vi "4.CVT Basic Writer.vi"() -> ()   [LabVIEW 2014]
uses:
  vi.lib/Q-WaveSystems/QwaveSys Raspberry Pi for LabVIEW Home-Education/CVT/_SubVIs/TypeDefs/cvt_Tag Configuration.ctl
  vi.lib/Q-WaveSystems/QwaveSys Raspberry Pi for LabVIEW Home-Education/CVT/_SubVIs/TypeDefs/cvt_Data Types.ctl
  vi.lib/Q-WaveSystems/QwaveSys Raspberry Pi for LabVIEW Home-Education/QwaveSys Raspberry Pi Library.lvlib
panel:
  out "Variable Name":string
  in  "stop":bool
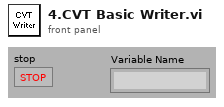
[diagram p1: front panel]
types:
  T1 = typedef "QwaveSys Raspberry Pi Library.lvlib/cvt_Tag Configuration.ctl" = cluster{"Name":string, "Data Type":T2, "Array":bool, "Size":u32, "Default":string, "Enum":string[], "Description":string}
  T2 = typedef "QwaveSys Raspberry Pi Library.lvlib/cvt_Data Types.ctl" = enum16{"Bool", "U8", "I32", "Double", "String", "Enum"}
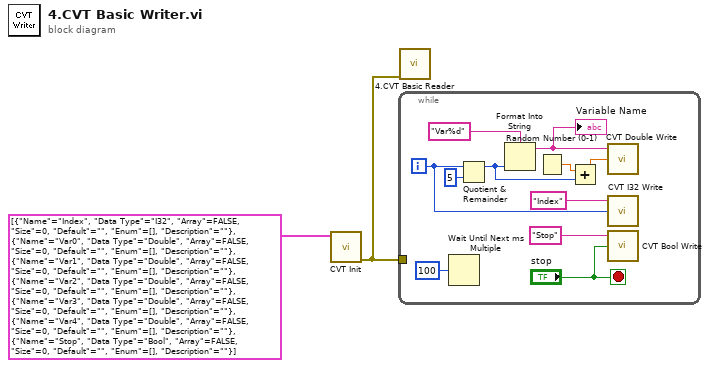
[diagram p0: block diagram]
diagram:
  n1 = call "CVT Init.vi"("Tag List"=T1[] [{"Name"="Index", "Data Type"=enum."I32", "Array"=FALSE, "Size"=0, "Default"="", "Enum"=[], "Description"=""}, {"Name"="Var0", "Data Type"=enum."Double", "Array"=FALSE, "Size"=0, "Default"="", "Enum"=[], "Description"=""}, {"Name"="Var1", "Data Type"=enum."Double", "Array"=FALSE, "Size"=0, "Default"="", "Enum"=[], "Description"=""}, {"Name"="Var2", "Data Type"=enum."Double", "Array"=FALSE, "Size"=0, "Default"="", "Enum"=[], "Description"=""}, {"Name"="Var3", "Data Type"=enum."Double", "Array"=FALSE, "Size"=0, "Default"="", "Enum"=[], "Description"=""}, {"Name"="Var4", "Data Type"=enum."Double", "Array"=FALSE, "Size"=0, "Default"="", "Enum"=[], "Description"=""}, {"Name"="Stop", "Data Type"=enum."Bool", "Array"=FALSE, "Size"=0, "Default"="", "Enum"=[], "Description"=""}]) -> ("error out"=w1:errorcluster)  [unwired: 1 in, 9 out]
  n2 = while {
    tunnel: w1 -> [_]
    i -> [w6]
    stop <- "stop" stop-if-true
    n3 = Wait Until Next ms Multiple(millisecond multiple=u32 100) -> ()  [unwired: 1 out]
    n4 = Quotient & Remainder(x=w6, y=5) -> (x-y*floor(x/y)=w3:i32)  [unwired: 1 out]
    n5 = Format Into String(format string="Var%d", w3) -> (resulting string=w9:string)  [unwired: 2 in, 1 out]
    "Variable Name" <- w9
    n6 = Random Number (0-1)() -> (number: 0 to 1=w5:dbl)
    n7 = Add(x=w5, y=w3) -> (x+y=w4:dbl)
    n8 = call "CVT Double Write.vi"("Value"=w4, "Tag Name"=w9) -> ()  [unwired: 1 in, 3 out]
    n9 = call "CVT I32 Write.vi"("Value"=w6, "Tag Name"="Index") -> ()  [unwired: 1 in, 3 out]
    n10 = call "CVT Bool Write.vi"("Value"="stop", "Tag Name"="Stop") -> ()  [unwired: 1 in, 3 out]
  }
  n11 = call "4.CVT Basic Reader.vi"("error in (no error)"=w1) -> ()  [unwired: 11 out]
